vi "InstruSweepControl_DP_ver1.0.vi"(3 "Run Index":i32, 6 "error in":errorcluster, 7 "output cluster":T1={"Main Sweep"=0, "Steps Config:"={"total points:"=0, "Step Delay (s)"=0.0, "Ini Delay (s)"=0.0, "# of steps:"=0}, "Temperature Control (ITC 503):"={"GPIB ADR"=0, "Change Heater?"={"Heater?"=FALSE, "Heater"=0}, "Change Temp?"={"Change T?"=FALSE, "Set T (K)"=0.0}, "Cluster"={"Heat Auto?"=FALSE, "Manual Heat?"=FALSE, "Heater (%)"=0.0}, "Change PID?"={"Change PID?"=FALSE, "P"=0.0, "I"=0.0, "D"=0.0}, "Change Para?"=FALSE, "Sensor"=1}, "Temperature Control (LS 340):"={"GPIB ADR"=0, "From (K)"=0.0, "To (K)"=0.0, "Rate (K/min)"=0.0, "Delta T (0.08K)"=0.0, "Temp. Header"="", "T Display Control"={"Ch B"=FALSE, "Ch C"=FALSE, "Ch D"=FALSE}}, "Magnet Control (IPS 120-10)"={"Action"=0, "Standby (s)"=0.0, "Heater on (s)"=0.0, "Sweep Setup "=[], "GPIB ADR"=0, "Change Para?"=FALSE}, "Keithley 6221 :"=[], "Measuring Instruments : "=[], "Lock-In SR7265 :"=[], "Deascription of \nthis measurement"="", "Instruments Config:"=[], "LS372 Bridge : 2"=[{"GPIB"=0, "Excitation"=0, "Autorange?"=FALSE, "Range"=0, "Current"=0, "Voltage"=0, "DataHeader"="Rx;Ry"}], "Magnet Control (CS4) 2"={"Action"=1, "Standby (s)"=0.0, "Heater on (s)"=300.0, "Sweep Setup "=[], "GPIB ADR"=0, "Change Para?"=FALSE}} {"Magnet Control (CS4) 2"."GPIB ADR" items=["None"=0, "25"=25]; "Magnet Control (CS4) 2"."Sweep Setup"."Rate in Range (T/min)" min=0.001 max=0.5 step=0.001; "Magnet Control (CS4) 2"."Sweep Setup"."Hold(min)" min=0.0; "Magnet Control (CS4) 2"."Sweep Setup"."Set Point (T)" min=-9.0 max=9.0 step=0.001; "Magnet Control (CS4) 2"."Action" items=["Up", "Down", "Pause", "Zero"]; "LS372 Bridge : 2"."Voltage" items=["2.00 uV"=1, "6.32 uV"=2, "20.0 uV"=3, "63.2 uV"=4, "200 uV"=5, "632 uV"=6, "2.0 mV"=7, "6.32 mV"=8]; "LS372 Bridge : 2"."Current" items=["1.00 pA"=1, "3.16 pA"=2, "10.0 pA"=3, "31.6 pA"=4, "100 pA"=5, "316 pA"=6, "1.00 nA"=7, "3.16 nA"=8, "10 nA"=9, "31.6 nA"=10, "100 nA"=11, "316 nA"=12, "1.00 uA"=13, "3.16 uA"=14, "10.0 uA"=15, "31.6 uA"=16, "100 uA"=17, "316 uA"=18, "1.00 mA"=19, "3.16 mA"=20, "10.0 mA"=21, "31.6 mA"=22]; "LS372 Bridge : 2"."Range" items=["2.0 m"=1, "6.32 m"=2, "20.0 m"=3, "63.2 m"=4, "200 m"=5, "632 m"=6, "2.00"=7, "6.32"=8, "20.0"=9, "63.2"=10, "200"=11, "632"=12, "2.00 k"=13, "6.32 k"=14, "20.0 k"=15, "63.2 k"=16, "200 k"=17, "632 k"=18, "2.00 M"=19, "6.32 M"=20, "20.0 M"=21, "63.2 M"=22]; "LS372 Bridge : 2"."Excitation" items=["Voltage", "Current"]; "LS372 Bridge : 2"."GPIB" items=["None"=0, "9"=9]; "Main Sweep" items=["Time", "DC Current", "Delta Current", "Pulse Delta Current", "Sine Current", "Lock-in Vosc"]; "Temperature Control (ITC 503):"."Sensor" items=["T2", "T3"]; "Magnet Control (IPS 120-10)"."Action" items=["Hold", "To Set point", "To Zero", "Clamp"]; "Keithley 6221 :"."Sweep Mode" items=["Linear", "Log", "Exp", "Inverse", "Manual"]}, 8 "2D Array of DC Source or Lock-In Ctrl Run Cluster":cluster{"GPIB ADR":u16, "DC St. Pt.":dbl}[][](array[cluster]), 9 "Stay duration pts":dbl[](array[numeric])) -> (0 "error out":errorcluster, 1 "output cluster 2":T1={"Main Sweep"=0, "Steps Config:"={"total points:"=0, "Step Delay (s)"=0.0, "Ini Delay (s)"=0.0, "# of steps:"=0}, "Temperature Control (ITC 503):"={"GPIB ADR"=0, "Change Heater?"={"Heater?"=FALSE, "Heater"=0}, "Change Temp?"={"Change T?"=FALSE, "Set T (K)"=0.0}, "Cluster"={"Heat Auto?"=FALSE, "Manual Heat?"=FALSE, "Heater (%)"=0.0}, "Change PID?"={"Change PID?"=FALSE, "P"=0.0, "I"=0.0, "D"=0.0}, "Change Para?"=FALSE, "Sensor"=1}, "Temperature Control (LS 340):"={"GPIB ADR"=0, "From (K)"=0.0, "To (K)"=0.0, "Rate (K/min)"=0.0, "Delta T (0.08K)"=0.0, "Temp. Header"="", "T Display Control"={"Ch B"=FALSE, "Ch C"=FALSE, "Ch D"=FALSE}}, "Magnet Control (IPS 120-10)"={"Action"=0, "Standby (s)"=0.0, "Heater on (s)"=0.0, "Sweep Setup "=[], "GPIB ADR"=0, "Change Para?"=FALSE}, "Keithley 6221 :"=[], "Measuring Instruments : "=[], "Lock-In SR7265 :"=[], "Deascription of \nthis measurement"="", "Instruments Config:"=[], "LS372 Bridge : 2"=[{"GPIB"=0, "Excitation"=0, "Autorange?"=FALSE, "Range"=0, "Current"=0, "Voltage"=0, "DataHeader"="Rx;Ry"}], "Magnet Control (CS4) 2"={"Action"=1, "Standby (s)"=0.0, "Heater on (s)"=300.0, "Sweep Setup "=[], "GPIB ADR"=0, "Change Para?"=FALSE}} {"Magnet Control (CS4) 2"."GPIB ADR" items=["None"=0, "25"=25]; "Magnet Control (CS4) 2"."Sweep Setup"."Rate in Range (T/min)" min=0.001 max=0.5 step=0.001; "Magnet Control (CS4) 2"."Sweep Setup"."Hold(min)" min=0.0; "Magnet Control (CS4) 2"."Sweep Setup"."Set Point (T)" min=-9.0 max=9.0 step=0.001; "Magnet Control (CS4) 2"."Action" items=["Up", "Down", "Pause", "Zero"]; "LS372 Bridge : 2"."Voltage" items=["2.00 uV"=1, "6.32 uV"=2, "20.0 uV"=3, "63.2 uV"=4, "200 uV"=5, "632 uV"=6, "2.0 mV"=7, "6.32 mV"=8]; "LS372 Bridge : 2"."Current" items=["1.00 pA"=1, "3.16 pA"=2, "10.0 pA"=3, "31.6 pA"=4, "100 pA"=5, "316 pA"=6, "1.00 nA"=7, "3.16 nA"=8, "10 nA"=9, "31.6 nA"=10, "100 nA"=11, "316 nA"=12, "1.00 uA"=13, "3.16 uA"=14, "10.0 uA"=15, "31.6 uA"=16, "100 uA"=17, "316 uA"=18, "1.00 mA"=19, "3.16 mA"=20, "10.0 mA"=21, "31.6 mA"=22]; "LS372 Bridge : 2"."Range" items=["2.0 m"=1, "6.32 m"=2, "20.0 m"=3, "63.2 m"=4, "200 m"=5, "632 m"=6, "2.00"=7, "6.32"=8, "20.0"=9, "63.2"=10, "200"=11, "632"=12, "2.00 k"=13, "6.32 k"=14, "20.0 k"=15, "63.2 k"=16, "200 k"=17, "632 k"=18, "2.00 M"=19, "6.32 M"=20, "20.0 M"=21, "63.2 M"=22]; "LS372 Bridge : 2"."Excitation" items=["Voltage", "Current"]; "LS372 Bridge : 2"."GPIB" items=["None"=0, "9"=9]; "Main Sweep" items=["Time", "DC Current", "Delta Current", "Pulse Delta Current", "Sine Current", "Lock-in Vosc"]; "Temperature Control (ITC 503):"."Sensor" items=["T2", "T3"]; "Magnet Control (IPS 120-10)"."Action" items=["Hold", "To Set point", "To Zero", "Clamp"]; "Keithley 6221 :"."Sweep Mode" items=["Linear", "Log", "Exp", "Inverse", "Manual"]}, 2 "Run Stop?":bool, 5 "Const I output":dbl[](array[numeric]))   [LabVIEW 2012]
panel:
  out "Set pt change Flags":bool[](array[boolean])
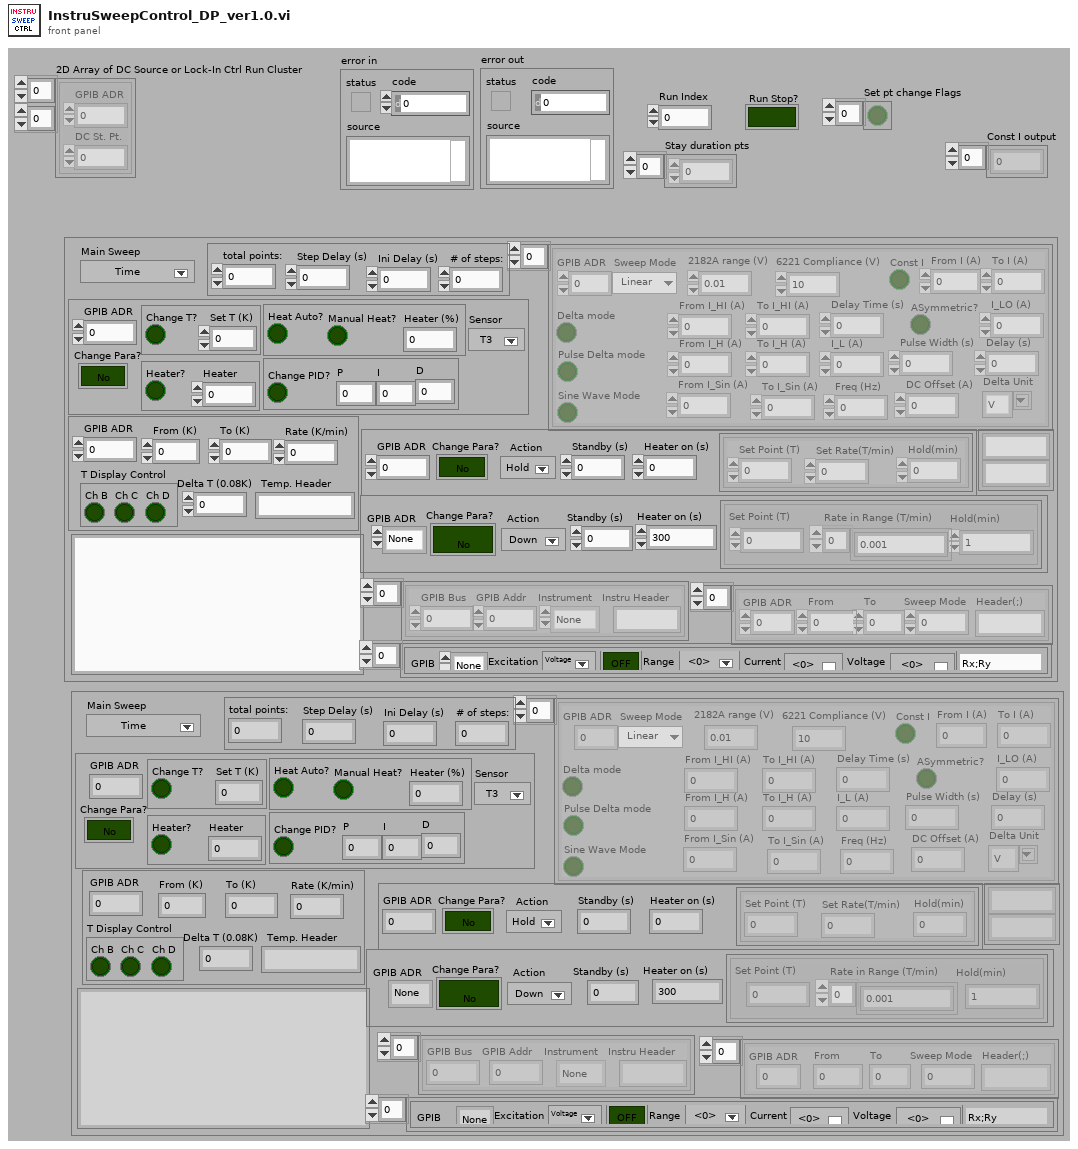
[diagram p1: front panel]
types:
  T1 = cluster{"Main Sweep":u8, "Steps Config:":cluster{"total points:":u32, "Step Delay (s)":dbl, "Ini Delay (s)":dbl, "# of steps:":u32}, "Temperature Control (ITC 503):":cluster{"GPIB ADR":u16, "Change Heater?":cluster{"Heater?":bool, "Heater":u8}, "Change Temp?":cluster{"Change T?":bool, "Set T (K)":dbl}, "Cluster":cluster{"Heat Auto?":bool, "Manual Heat?":bool, "Heater (%)":dbl}, "Change PID?":cluster{"Change PID?":bool, "P":dbl, "I":dbl, "D":dbl}, "Change Para?":bool, "Sensor":u16}, "Temperature Control (LS 340):":cluster{"GPIB ADR":u16, "From (K)":dbl, "To (K)":dbl, "Rate (K/min)":dbl, "Delta T (0.08K)":dbl, "Temp. Header":string, "T Display Control":cluster{"Ch B":bool, "Ch C":bool, "Ch D":bool}}, "Magnet Control (IPS 120-10)":cluster{"Action":u16, "Standby (s)":dbl, "Heater on (s)":dbl, "Sweep Setup ":cluster{"Set Point (T)":dbl, "Set Rate(T/min)":dbl, "Hold(min)":dbl}[], "GPIB ADR":u16, "Change Para?":bool}, "Keithley 6221 :":cluster{"Delta mode":bool, "Const I":bool, "Pulse Delta mode":bool, "Sine Wave Mode":bool, "From I_HI (A)":dbl, "From I (A)":dbl, "I_LO (A)":dbl, "From I_H (A)":dbl, "I_L (A)":dbl, "Freq (Hz)":dbl, "From I_Sin (A)":dbl, "DC Offset (A)":dbl, "Delay Time (s)":dbl, "Pulse Width (s)":dbl, "Delay (s)":dbl, "To I (A)":dbl, "ASymmetric?":bool, "To I_HI (A)":dbl, "To I_H (A)":dbl, "To I_Sin (A)":dbl, "GPIB ADR":u16, "Sweep Mode":u8, "Delta Unit":string, "2182A range (V)":dbl, "6221 Compliance (V)":dbl}[], "Measuring Instruments : ":cluster{"GPIB Bus":dbl, "GPIB Addr":dbl, "Instrument":enum16{"None", "HP34401DMM", "Lockin 7265", "HP3456/7A", "HP3478A", "HP3325FG", "Keithley2182A"}, "Instru Header":string}[], "Lock-In SR7265 :":cluster{"GPIB ADR":u16, "From":dbl, "To":dbl, "Header(;)":string, "Sweep Mode":u8}[], "Deascription of \nthis measurement":string, "Instruments Config:":string[][], "LS372 Bridge : 2":cluster{"GPIB":u16, "Excitation":u16, "Autorange?":bool, "Range":u16, "Current":u16, "Voltage":u16, "DataHeader":string}[], "Magnet Control (CS4) 2":cluster{"Action":u16, "Standby (s)":dbl, "Heater on (s)":dbl, "Sweep Setup ":cluster{"Set Point (T)":dbl, "Hold(min)":dbl, "Rate in Range (T/min)":dbl[]}[], "GPIB ADR":u16, "Change Para?":bool}}
  T2 = cluster{"total points:":u32, "Step Delay (s)":dbl, "Ini Delay (s)":dbl, "# of steps:":u32}
  T3 = cluster{"Delta mode":bool, "Const I":bool, "Pulse Delta mode":bool, "Sine Wave Mode":bool, "From I_HI (A)":dbl, "From I (A)":dbl, "I_LO (A)":dbl, "From I_H (A)":dbl, "I_L (A)":dbl, "Freq (Hz)":dbl, "From I_Sin (A)":dbl, "DC Offset (A)":dbl, "Delay Time (s)":dbl, "Pulse Width (s)":dbl, "Delay (s)":dbl, "To I (A)":dbl, "ASymmetric?":bool, "To I_HI (A)":dbl, "To I_H (A)":dbl, "To I_Sin (A)":dbl, "GPIB ADR":u16, "Sweep Mode":u8, "Delta Unit":string, "2182A range (V)":dbl, "6221 Compliance (V)":dbl}[]
  T4 = cluster{"Delta mode":bool, "Const I":bool, "Pulse Delta mode":bool, "Sine Wave Mode":bool, "From I_HI (A)":dbl, "From I (A)":dbl, "I_LO (A)":dbl, "From I_H (A)":dbl, "I_L (A)":dbl, "Freq (Hz)":dbl, "From I_Sin (A)":dbl, "DC Offset (A)":dbl, "Delay Time (s)":dbl, "Pulse Width (s)":dbl, "Delay (s)":dbl, "To I (A)":dbl, "ASymmetric?":bool, "To I_HI (A)":dbl, "To I_H (A)":dbl, "To I_Sin (A)":dbl, "GPIB ADR":u16, "Sweep Mode":u8, "Delta Unit":string, "2182A range (V)":dbl, "6221 Compliance (V)":dbl}
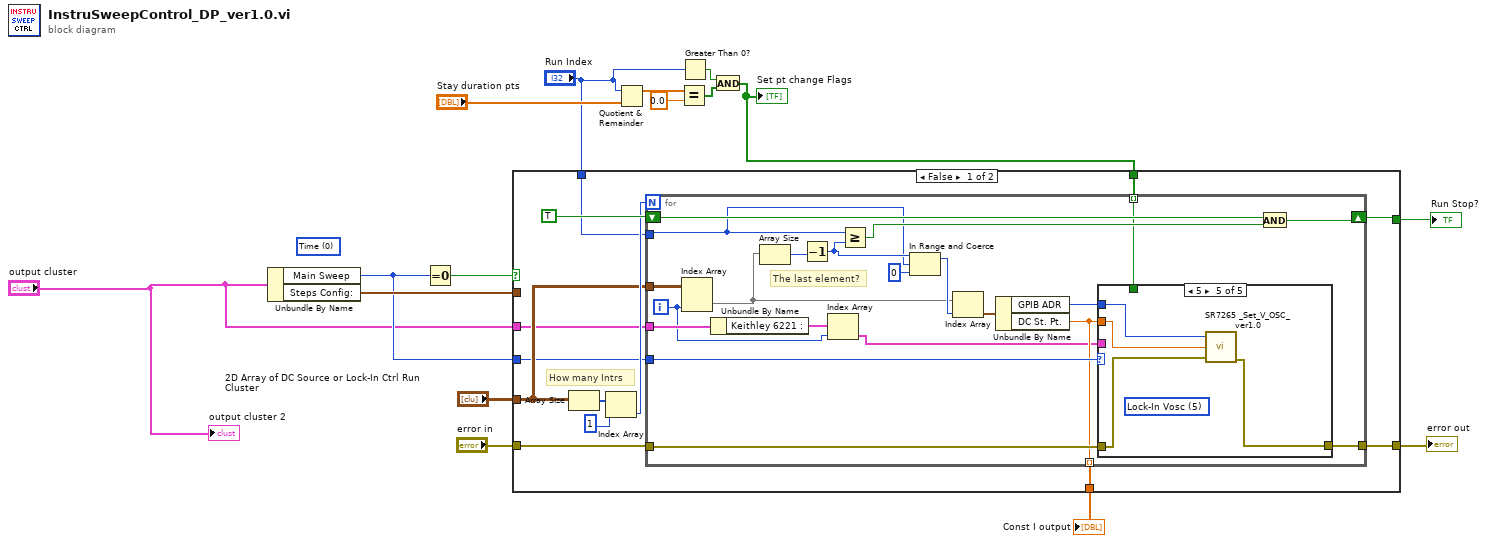
[diagram p0: block diagram]
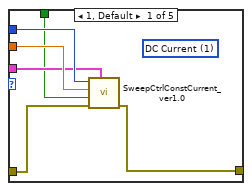
[diagram p2: hidden frame]
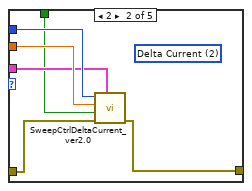
[diagram p3: hidden frame]
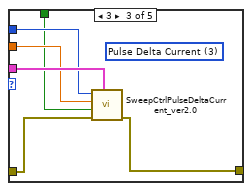
[diagram p4: hidden frame]
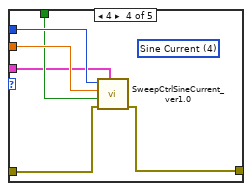
[diagram p5: hidden frame]
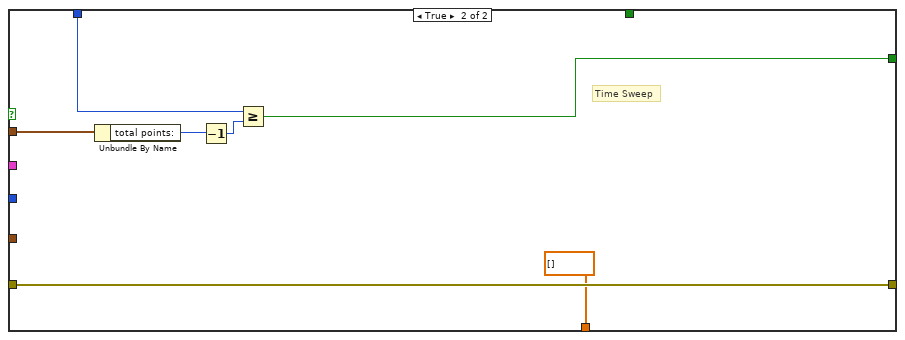
[diagram p6: hidden frame]
diagram:
  (unwired) u8 0 items=["Time", "DC Current", "Delta Current", "Pulse Delta Current", "Sine Current", "Lock-In Vosc"] ("Main Sweep")
  n1 = Unbundle By Name("output cluster") -> ("Main Sweep"=w10:u8, "Steps Config:"=w16:T2)
  n2 = Equal To 0?(x=w10) -> (x = 0?=w11:bool)
  n3 = Quotient & Remainder(x="Run Index", y="Stay duration pts") -> (x-y*floor(x/y)=w9:dbl[])  [unwired: 1 out]
  n4 = Equal?(x=w9, y=0.0) -> (x = y?=w4:bool[])
  n5 = Greater Than 0?(x="Run Index") -> (x > 0?=w5:bool)
  n6 = And(x=w5, y=w4) -> (x .and. y?=w3:bool[])
  "Set pt change Flags" <- w3
  n7 = case shown="False" w11 {
    tunnel: w16 -> [_ w85]
    tunnel: "Run Index" -> [w23 w82]
    tunnel: [w20 w81] -> w15
    tunnel: "error in" -> [w24 w80]
    tunnel: [w21 w80] -> w13
    tunnel: "2D Array of DC Source or Lock-In Ctrl Run Cluster" -> [w25 _]
    tunnel: w10 -> [w22 _]
    tunnel: w3 -> [w19 _]
    tunnel: [w18 dbl[] []] -> w2
    tunnel: "output cluster" -> [w17 _]
    frame False {
      # "How many Intrs"
      n8 = Array Size(array=w25) -> (size(s)=w27:i32[])
      n9 = Index Array(array=w27, index=1) -> (element=w26:i32)
      n10 = for {
        N: w26 -> [_]
        shift-right: [w49] -> w20
        shift-left: TRUE -> [w50]
        tunnel: w25 -> [w48]
        tunnel: w24 -> [w39]
        tunnel: w23 -> [w44]
        tunnel: w22 -> [w41]
        tunnel: [w38] -> w21
        tunnel: w19 -> [w35] mode=indexing
        tunnel: [w34] -> w18 mode=indexing
        tunnel: w17 -> [w33]
        i -> [w31]
        # "The last element?"
        n11 = Index Array(array=w48, index (col)=w31) -> (element=w36:cluster{"GPIB ADR":u16, "DC St. Pt.":dbl}[])  [unwired: 1 in]
        n12 = Unbundle By Name(w33) -> ("Keithley 6221 :"=w32:T3)
        n13 = Array Size(array=w36) -> (size(s)=w47:i32)
        n14 = Decrement(x=w47) -> (x-1=w45:i32)
        n15 = Index Array(array=w32, index=w31) -> (element=w30:T4)
        n16 = Greater Or Equal?(x=w44, y=w45) -> (x >= y?=w46:bool)
        n17 = In Range and Coerce(upper limit=w45, x=w44, lower limit=0) -> (coerced(x)=w37:i32)  [unwired: 1 out]
        n18 = Index Array(array=w36, index=w37) -> (element=w42:cluster{"GPIB ADR":u16, "DC St. Pt.":dbl})
        n19 = Unbundle By Name(w42) -> ("GPIB ADR"=w40:u16, "DC St. Pt."=w34:dbl)
        n20 = case shown="5" w41 {
          tunnel: w40 -> [w56 w62 w67 w74 w75]
          tunnel: w34 -> [w55 w61 w66 w73 w76]
          tunnel: w39 -> [w52 w58 w64 w71 w78]
          tunnel: [w51 w57 w63 w70 w77] -> w38
          tunnel: w30 -> [w54 w60 w68 w69 _]
          tunnel: w35 -> [w53 w59 w65 w72 _]
          frame 1, Default {
            (unwired) u8 1 items=["Time", "DC Current", "Delta Current", "Pulse Delta Current", "Sine Current", "Lock-In Vosc"] ("Main Sweep")
            n21 = call "SweepCtrlConstCurrent_ver1.0.vi"("Keithley 6221"=w54, "error in (no error)"=w52, "Set pt change flag"=w53, "DC St. Pt."=w55, "GPIB ADR"=w56) -> ("error out"=w51:errorcluster)  [unwired: 6 in]
          }
          frame 2 {
            (unwired) u8 2 items=["Time", "DC Current", "Delta Current", "Pulse Delta Current", "Sine Current", "Lock-In Vosc"] ("Main Sweep")
            n22 = call "SweepCtrlDeltaCurrent_ver2.0.vi"("Keithley 6221"=w60, "error in (no error)"=w58, "Set pt change flag"=w59, "DC St. Pt."=w61, "GPIB ADR"=w62) -> ("error out"=w57:errorcluster)  [unwired: 6 in]
          }
          frame 3 {
            (unwired) u8 3 items=["Time", "DC Current", "Delta Current", "Pulse Delta Current", "Sine Current", "Lock-In Vosc"] ("Main Sweep")
            n23 = call "SweepCtrlPulseDeltaCurrent_ver2.0.vi"("Keithley 6221"=w68, "error in (no error)"=w64, "Set pt change flag"=w65, "DC St. Pt."=w66, "GPIB ADR"=w67) -> ("error out"=w63:errorcluster)  [unwired: 6 in]
          }
          frame 4 {
            (unwired) u8 4 items=["Time", "DC Current", "Delta Current", "Pulse Delta Current", "Sine Current", "Lock-In Vosc"] ("Main Sweep")
            n24 = call "SweepCtrlSineCurrent_ver1.0.vi"("Keithley 6221"=w69, "error in (no error)"=w71, "Set pt change flag"=w72, "DC St. Pt."=w73, "GPIB ADR"=w74) -> ("error out"=w70:errorcluster)  [unwired: 6 in]
          }
          frame 5 {
            (unwired) u8 5 items=["Time", "DC Current", "Delta Current", "Pulse Delta Current", "Sine Current", "Lock-In Vosc"] ("Main Sweep")
            n25 = call "SR7265 _Set_V_OSC_ver1.0.vi"("GPIB ADR"=w75, "Vosc Setpt"=w76, "error in"=w78) -> ("error out"=w77:errorcluster)  [unwired: 1 in, 2 out]
          }
        }
        n26 = And(x=w50, y=w46) -> (x .and. y?=w49:bool)
      }
    }
    frame True {
      # "Time Sweep"
      n27 = Unbundle By Name(w85) -> ("total points:"=w84:u32)
      n28 = Decrement(x=w84) -> (x-1=w83:u32)
      n29 = Greater Or Equal?(x=w82, y=w83) -> (x >= y?=w81:bool)
    }
  }
  "Run Stop?" <- w15
  "error out" <- w13
  "Const I output" <- w2
  "output cluster 2" <- "output cluster"
